vi "闹钟（每分）.vi"() -> (7 "TimeReached":bool)   [LabVIEW 2012]
panel:
  out "分":i32
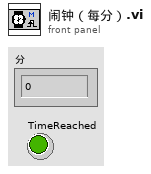
[diagram p1: front panel]
types:
  T1 = typedef "LVDateTimeRec.ctl" = cluster{"秒数的小数部分":dbl, "秒":i32, "分":i32, "时":i32, "日":i32, "月":i32, "年":i32, "天数（周）":i32, "天数（年）":i32, "DST":i32}
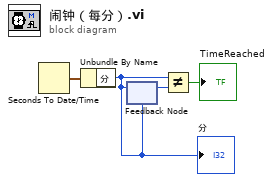
[diagram p0: block diagram]
diagram:
  n1 = Seconds To Date/Time() -> (date time rec=w4:T1)  [unwired: 2 in]
  n2 = Unbundle By Name(w4) -> ("分"=w1:i32)
  "分" <- w1
  n3 = feedback #1(w1) -> (w3:i32)
  n4 = feedback-in #1(w1) -> ()
  n5 = Not Equal?(x=w1, y=w3) -> (x != y?=→"TimeReached":bool)
